vi "Menu Activation.vi"(8 "error in (no error)":errorcluster, 11 "HIJ 4 Alignment Cams App in":refnum<class "HIJ 4 Alignment Cams App.lvclass">) -> (0 "error out":errorcluster, 3 "HIJ 4 Alignment Cams App out":refnum<class "HIJ 4 Alignment Cams App.lvclass">)   [LabVIEW 2014, in "HIJ 4 Alignment Cams App.lvlib" / "HIJ 4 Alignment Cams App.lvclass"]
uses:
  HIJ 4 Alignment Cams App.lvclass
  HIJ 4 Alignment Cams App.lvclass/HIJ 4 Alignment Cams App.ctl
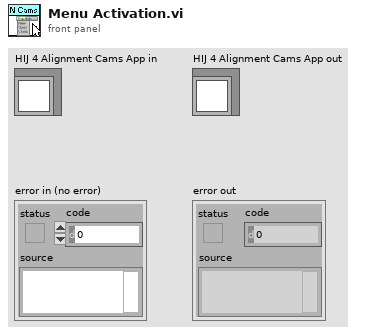
[diagram p1: front panel]
types:
  T1 = typedef "HIJ 4 Alignment Cams App.lvlib/HIJ 4 Alignment Cams App.lvclass/CamAppInfo.ctl" = cluster{"Camera":T2, "App enq":refnum<class "Message Enqueuer.lvclass">, "SubPnl Refnum":refnum<vi>}
  T2 = typedef "IMAQdx.ctl" = refnum<k21>
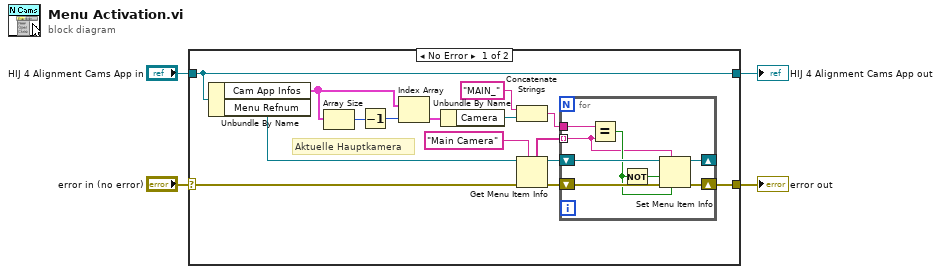
[diagram p0: block diagram]
diagram:
  n1 = case shown="No Error" "error in (no error)" {
    selector: "error in (no error)" -> [w8 w29]
    tunnel: [w7 w29] -> w3
    tunnel: [w19 w28] -> w1
    tunnel: "HIJ 4 Alignment Cams App in" -> [w19 w28]
    frame No Error {
      # "Aktuelle Hauptkamera"
      n2 = Unbundle By Name(w19) -> ("Cam App Infos"=w16:T1[], "Menu Refnum"=w5:refnum<k9>)
      n3 = Array Size(array=w16) -> (size(s)=w17:i32)
      n4 = Decrement(x=w17) -> (x-1=w15:i32)
      n5 = Index Array(array=w16, index=w15) -> (element=w14:T1)
      n6 = Unbundle By Name(w14) -> ("Camera"=w6:T2)
      n7 = Concatenate Strings("MAIN_" ("string"), w6) -> (w11:string)
      n8 = Get Menu Item Info(7:"Main Camera" ("item tag"), 8:w8, 11:w5) -> (0:w9:errorcluster, 3:w12:refnum<k9>, 5:w10:string[])  [unwired: 4 out]
      n9 = for {
        tunnel: w11 -> [w23]
        tunnel: w10 -> [w20] mode=indexing
        shift-right: [w25] -> w7
        shift-left: w9 -> [w26]
        shift-right: [w24] -> _
        shift-left: w12 -> [w27]
        n10 = Equal?(x=w23, y=w20) -> (x = y?=w22:bool)
        n11 = Not(x=w22) -> (.not. x?=w21:bool)
        n12 = Set Menu Item Info(6:w22, 7:w20, 8:w26, 9:w21, 11:w27) -> (0:w25:errorcluster, 3:w24:refnum<k9>)  [unwired: 2 in]
      }
    }
    frame Error {
    }
  }
  "error out" <- w3
  "HIJ 4 Alignment Cams App out" <- w1
